vi "DeleteSection.vi"(6 "Function":enum16{"Default"}(ring), 8 "error in (no error)":errorcluster, 9 "Any Point?":bool, 10 "Range":T1, 11 "All Lines":T2) -> (0 "error out":errorcluster, 3 "output array":T2)   [LabVIEW 2014]
uses:
  Libraries/Map Data Folder/All-Lines.ctl
  Libraries/Map Data Folder/LineCluster.ctl
  Libraries/Map Data Folder/LineConnection.ctl
  Libraries/Map Data Folder/Map Data.lvlib
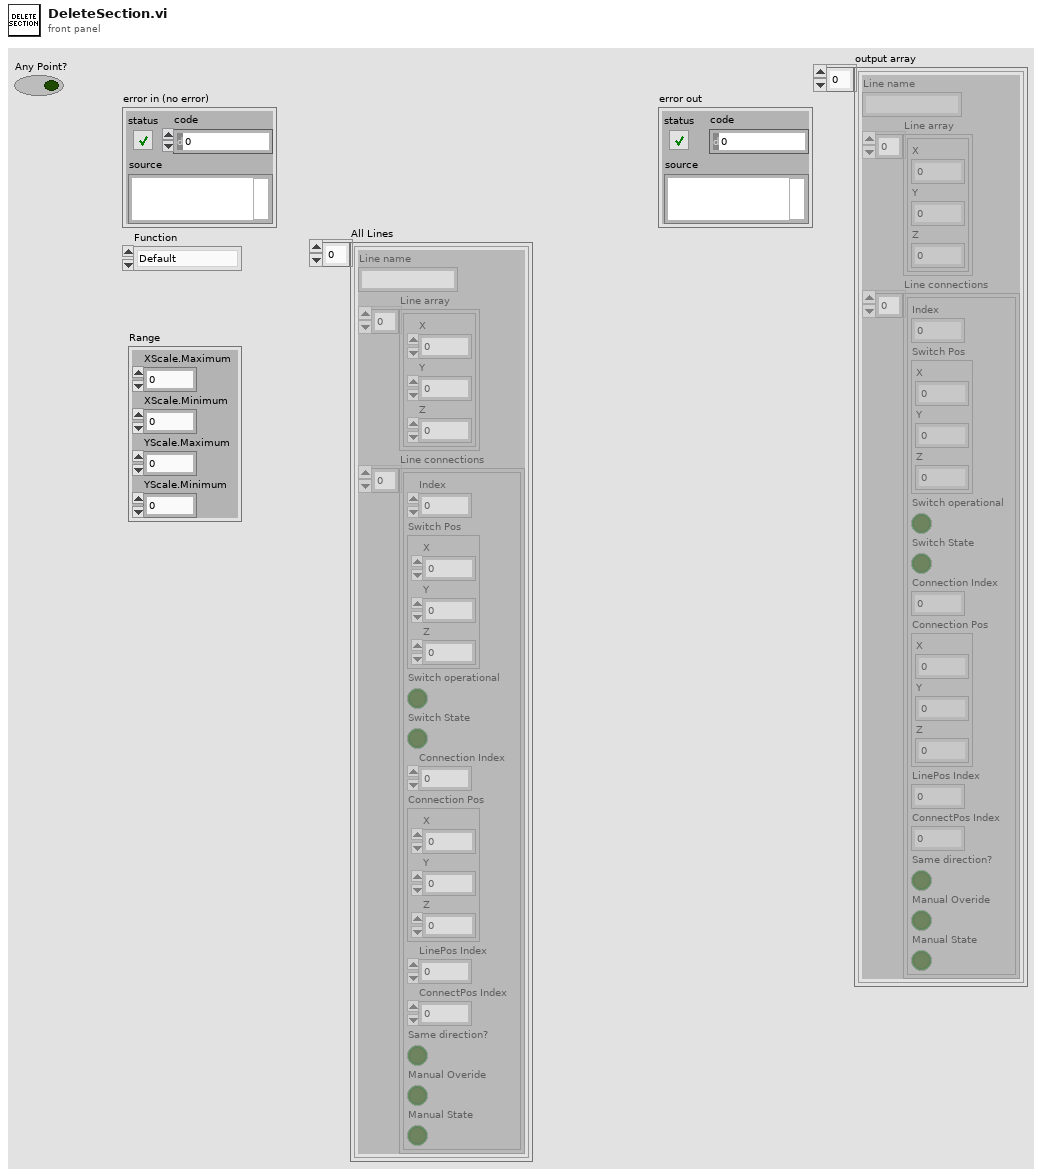
[diagram p1: front panel]
types:
  T1 = cluster{"XScale.Maximum":dbl, "XScale.Minimum":dbl, "YScale.Maximum":dbl, "YScale.Minimum":dbl}
  T2 = typedef "Map Data.lvlib/All-Lines.ctl" = T3[]
  T3 = typedef "Map Data.lvlib/LineCluster.ctl" = cluster{"Line name":string, "Line array":cluster{"X":dbl, "Y":dbl, "Z":dbl}[], "Line connections":T4[]}
  T4 = typedef "LineConnection.ctl" = cluster{"Index":i32, "Switch Pos":cluster{"X":dbl, "Y":dbl, "Z":dbl}, "Switch operational":bool, "Switch State":bool, "Connection Index":i32, "Connection Pos":cluster{"X":dbl, "Y":dbl, "Z":dbl}, "LinePos Index":i32, "ConnectPos Index":i32, "Same direction?":bool, "Manual Overide":bool, "Manual State":bool}
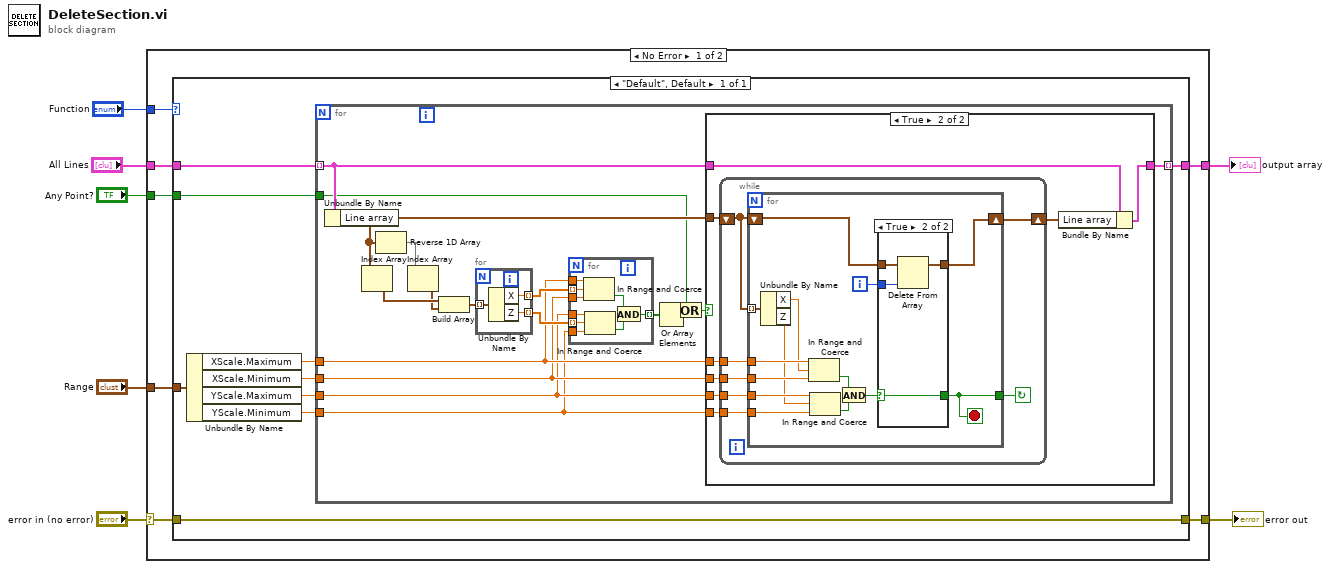
[diagram p0: block diagram]
diagram:
  n1 = case shown="No Error" "error in (no error)" {
    selector: "error in (no error)" -> [w13 w89]
    tunnel: [w14 w89] -> w7
    tunnel: "Function" -> [w12 _]
    tunnel: "All Lines" -> [w11 w90]
    tunnel: [w10 w90] -> w3
    tunnel: "Range" -> [w9 _]
    tunnel: "Any Point?" -> [w8 _]
    frame No Error {
      n2 = case shown="\"Default\", Default" w12 {
        tunnel: [w23] -> w14
        tunnel: w13 -> [w23]
        tunnel: w11 -> [w21]
        tunnel: [w22] -> w10
        tunnel: w9 -> [w20]
        tunnel: w8 -> [w15]
        frame "Default", Default {
          n3 = Unbundle By Name(w20) -> ("XScale.Maximum"=w19:dbl, "XScale.Minimum"=w18:dbl, "YScale.Maximum"=w17:dbl, "YScale.Minimum"=w16:dbl)
          n4 = for {
            tunnel: [w28] -> w22 mode=indexing
            tunnel: w21 -> [w27] mode=indexing
            tunnel: w19 -> [w32]
            tunnel: w18 -> [w31]
            tunnel: w17 -> [w30]
            tunnel: w16 -> [w29]
            tunnel: w15 -> [w24]
            n5 = Unbundle By Name(w27) -> ("Line array"=w26:cluster{"X":dbl, "Y":dbl, "Z":dbl}[])
            n6 = Index Array(array=w26) -> (element=w39:cluster{"X":dbl, "Y":dbl, "Z":dbl})  [unwired: 1 in]
            n7 = Reverse 1D Array(array=w26) -> (reversed array=w40:cluster{"X":dbl, "Y":dbl, "Z":dbl}[])
            n8 = Index Array(array=w40) -> (element=w38:cluster{"X":dbl, "Y":dbl, "Z":dbl})  [unwired: 1 in]
            n9 = Build Array(w39, w38) -> (w37:cluster{"X":dbl, "Y":dbl, "Z":dbl}[])
            n10 = for {
              tunnel: w37 -> [w79] mode=indexing
              tunnel: [w78] -> w36 mode=indexing
              tunnel: [w77] -> w35 mode=indexing
              n11 = Unbundle By Name(w79) -> ("X"=w78:dbl, "Z"=w77:dbl)
            }
            n12 = for {
              tunnel: w32 -> [w88]
              tunnel: w31 -> [w87]
              tunnel: w30 -> [w86]
              tunnel: w29 -> [w85]
              tunnel: w36 -> [w84] mode=indexing
              tunnel: w35 -> [w83] mode=indexing
              tunnel: [w80] -> w34 mode=indexing
              n13 = In Range and Coerce(upper limit=w88, x=w84, lower limit=w87) -> (In Range?=w81:bool)  [unwired: 1 out]
              n14 = In Range and Coerce(upper limit=w86, x=w83, lower limit=w85) -> (In Range?=w82:bool)  [unwired: 1 out]
              n15 = And(x=w81, y=w82) -> (x .and. y?=w80:bool)
            }
            n16 = Or Array Elements(Boolean array=w34) -> (logical OR=w33:bool)
            n17 = Or(x=w24, y=w33) -> (x .or. y?=w25:bool)
            n18 = case shown="True" w25 {
              tunnel: w32 -> [_ w48]
              tunnel: w31 -> [_ w47]
              tunnel: w30 -> [_ w46]
              tunnel: w29 -> [_ w45]
              tunnel: [w41 w42] -> w28
              tunnel: w27 -> [w41 w43]
              tunnel: w26 -> [_ w49]
              frame False {
              }
              frame True {
                n19 = while {
                  tunnel: w48 -> [w56]
                  tunnel: w47 -> [w55]
                  tunnel: w46 -> [w54]
                  tunnel: w45 -> [w53]
                  shift-right: [w50] -> w44
                  shift-left: w49 -> [w52]
                  stop <- w51 continue-if-true
                  n20 = for {
                    tunnel: w52 -> [w64] mode=indexing
                    tunnel: w56 -> [w70]
                    tunnel: w55 -> [w69]
                    tunnel: w54 -> [w68]
                    tunnel: w53 -> [w67]
                    shift-right: [w62] -> w50
                    shift-left: w52 -> [w63]
                    tunnel: [w60] -> w51
                    i -> [w61]
                    stop <- w60 stop-if-true
                    n21 = Unbundle By Name(w64) -> ("X"=w65:dbl, "Z"=w66:dbl)
                    n22 = In Range and Coerce(upper limit=w70, x=w65, lower limit=w69) -> (In Range?=w58:bool)  [unwired: 1 out]
                    n23 = In Range and Coerce(upper limit=w68, x=w66, lower limit=w67) -> (In Range?=w59:bool)  [unwired: 1 out]
                    n24 = And(x=w58, y=w59) -> (x .and. y?=w57:bool)
                    n25 = case shown="True" w57 {
                      selector: w57 -> [w71 w73]
                      tunnel: w63 -> [w72 w76]
                      tunnel: [w72 w75] -> w62
                      tunnel: w61 -> [_ w74]
                      tunnel: [w71 w73] -> w60
                      frame False {
                      }
                      frame True {
                        n26 = Delete From Array(array=w76, index=w74) -> (array with subset deleted=w75:cluster{"X":dbl, "Y":dbl, "Z":dbl}[])  [unwired: 1 in, 1 out]
                      }
                    }
                  }
                }
                n27 = Bundle By Name(cluster=w43, "Line array"=w44) -> (w42:T3)
              }
            }
          }
        }
      }
    }
    frame Error {
    }
  }
  "error out" <- w7
  "output array" <- w3
